vi "Set-pane-status.vi"(8 "error in (no error)":errorcluster, 9 "Status":bool, 10 "Pane":T1, 11 "Panes in":T2) -> (0 "error out":errorcluster, 3 "Panes out":T2)   [LabVIEW 2013, in "HardwareCharacterization.lvlib" / "HC-UI.lvclass"]
uses:
  HC-UI.lvclass
  Panes-reference.ctl
  Pane-names.ctl
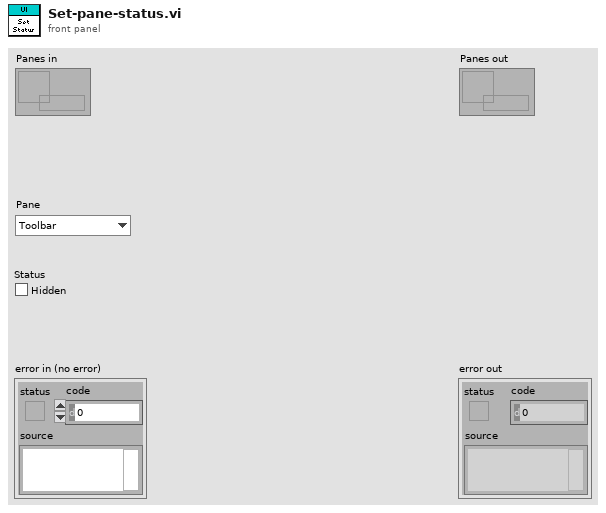
[diagram p1: front panel]
types:
  T1 = typedef "HardwareCharacterization.lvlib/HC-UI.lvclass/Pane-names.ctl" = enum16{"Toolbar", "Help bar", "Toolbar lower border", "Center panel", "Main panel", "Settings panel", "Status bar upper border", "General state bar", "Information bar"}
  T2 = typedef "HardwareCharacterization.lvlib/HC-UI.lvclass/Panes-reference.ctl" = refnum<data-value>
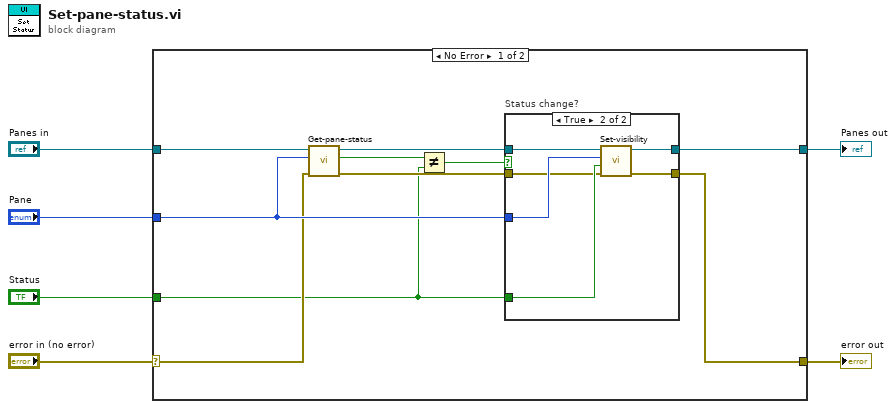
[diagram p0: block diagram]
diagram:
  n1 = case shown="No Error" "error in (no error)" {
    selector: "error in (no error)" -> [w11 w25]
    tunnel: [w14 w25] -> w5
    tunnel: [w15 w26] -> w3
    tunnel: "Panes in" -> [w16 w26]
    tunnel: "Pane" -> [w12 _]
    tunnel: "Status" -> [w7 _]
    frame No Error {
      n2 = call "Get-pane-status.vi"("error in (no error)"=w11, "Pane"=w12, "Panes in"=w16) -> ("error out"=w10:errorcluster, "Status"=w9:bool, "Panes out"=w13:T2)  [unwired: 6 in]
      n3 = Not Equal?(x=w9, y=w7) -> (x != y?=w8:bool)
      n4 = case "Status change?" shown="True" w8 {
        tunnel: [w17 w24] -> w15
        tunnel: [w18 w23] -> w14
        tunnel: w7 -> [_ w22]
        tunnel: w13 -> [w17 w21]
        tunnel: w12 -> [_ w20]
        tunnel: w10 -> [w18 w19]
        frame False {
        }
        frame True {
          n5 = call "Set-visibility.vi"("error in (no error)"=w19, "Visibility"=w22, "Pane"=w20, "Panes in"=w21) -> ("error out"=w23:errorcluster, "Panes out"=w24:T2)  [unwired: 6 in]
        }
      }
    }
    frame Error {
    }
  }
  "error out" <- w5
  "Panes out" <- w3
